vi "Bool to String.vi"(3 "Bool":bool) -> (1 "String":string)   [LabVIEW 2020, in "Vecto.lvlib"]
uses:
  Vecto.lvlib
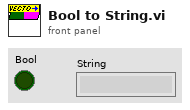
[diagram p1: front panel]
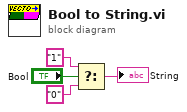
[diagram p0: block diagram]
diagram:
  n1 = Select(t="1", s="Bool", f="0") -> (s? t:f=→"String":string)
